vi "Time_to_String_Array.vi"(11 "String Array In":string[](array[string])) -> (3 "String Array Out":string[](array[string]))   [LabVIEW 2021]
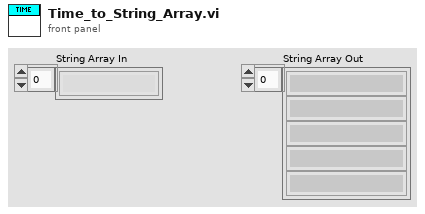
[diagram p1: front panel]
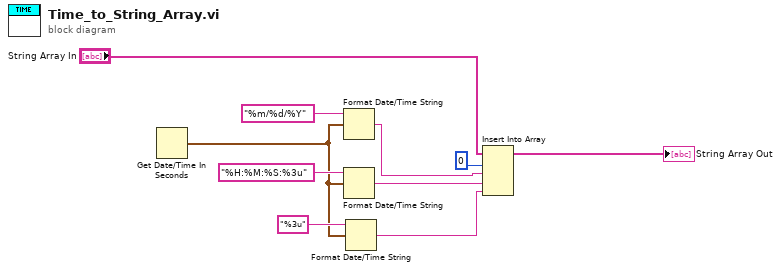
[diagram p0: block diagram]
diagram:
  n1 = Get Date/Time In Seconds() -> (seconds since 1Jan1904=w2:timestamp)
  n2 = Format Date/Time String(time format string (%c)="%m/%d/%Y", seconds (now)=w2) -> (date/time string=w8:string)  [unwired: 1 in]
  n3 = Format Date/Time String(time format string (%c)="%H:%M:%S:%3u", seconds (now)=w2) -> (date/time string=w9:string)  [unwired: 1 in]
  n4 = Format Date/Time String(time format string (%c)="%3u", seconds (now)=w2) -> (date/time string=w1:string)  [unwired: 1 in]
  n5 = Insert Into Array(array="String Array In", index=0, new element #1=w8, new element #2=w9, new element #3=w1) -> (→"String Array Out":string[])
